vi "Destructor.vi"(8 "error in (no error)":errorcluster, 11 "SingletonDVR In":refnum<data-value>) -> (0 "error out":errorcluster, 3 "Singleton.lvclass Out":refnum<class "Singleton.lvclass">)   [LabVIEW 2013, in "Singleton.lvclass"]
uses:
  Singleton.lvclass
panel:
  # "SingletonDestructor"
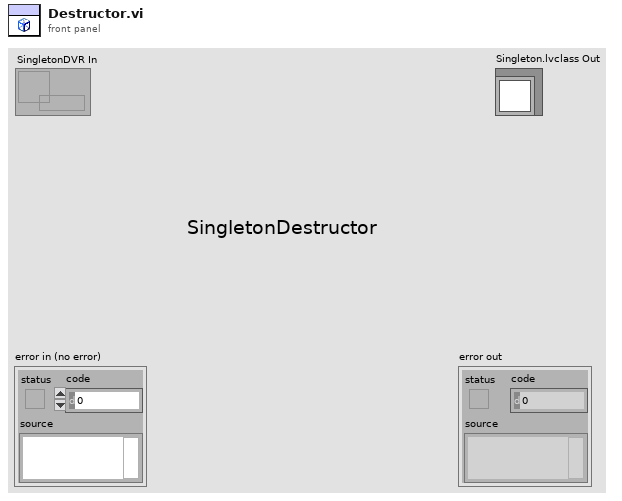
[diagram p1: front panel]
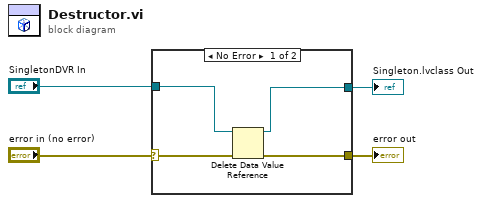
[diagram p0: block diagram]
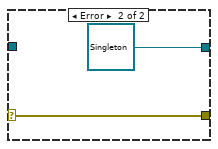
[diagram p2: hidden frame]
diagram:
  n1 = case shown="No Error" "error in (no error)" {
    selector: "error in (no error)" -> [w8 w10]
    tunnel: [w5 w10] -> w3
    tunnel: "SingletonDVR In" -> [w7 _]
    tunnel: [w6 refnum<class "Singleton.lvclass"> refnum ("Singleton in")] -> w1
    frame No Error {
      n2 = Delete Data Value Reference(data value reference=w7, error in=w8) -> (data value=w6:refnum<class "Singleton.lvclass">, error out=w5:errorcluster)
    }
    frame Error {
    }
  }
  "error out" <- w3
  "Singleton.lvclass Out" <- w1
